vi "configurePorts.vi"   [LabVIEW 2017]
uses:
  globalDevices.vi
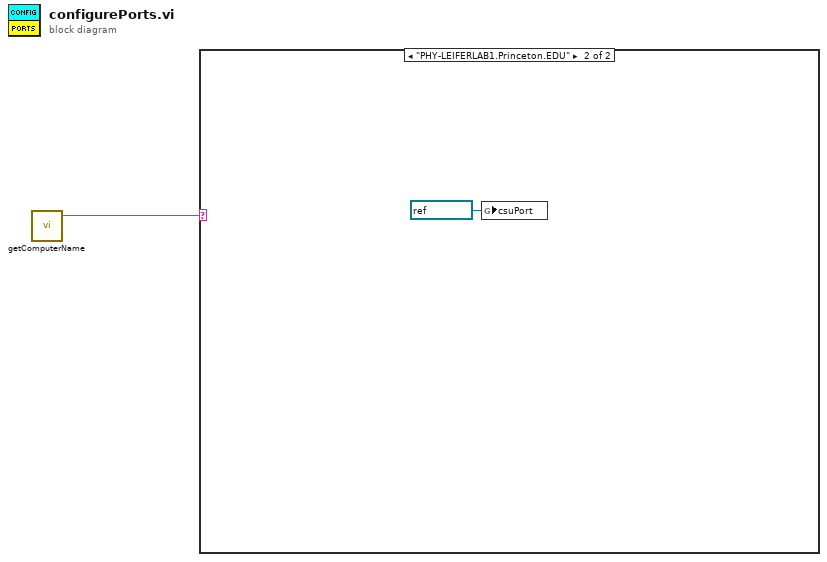
[diagram p0: block diagram]
diagram:
  n1 = call "getComputerName.vi"() -> ("full name"=w1:string)  [unwired: 1 in, 2 out]
  n2 = case shown="\"PHY-LEIFERLAB1.Princeton.EDU\"" w1 {
    frame "False", Default {
    }
    frame "PHY-LEIFERLAB1.Princeton.EDU" {
      n3 = global write "globalDevices.vi" "csuPort"(refnum<visa-resource-name> "COM1" ("csuPort")) -> ()
    }
  }
